vi "Execute Error Handling.vi"(8 "error in (no error)":errorcluster, 9 "Error":errorcluster, 10 "Error Level":T1, 11 "Interface Elevator in":refnum<class "Interface Elevator.lvclass">) -> (0 "error out":errorcluster, 3 "Interface Elevator out":refnum<class "Interface Elevator.lvclass">)   [LabVIEW 2022 SP3, in "Interface Elevator.lvclass"]
uses:
  Interface Elevator.lvclass
  Elevator Controller Actor/Elevator Controller Actor/Error Level.ctl
  Elevator Controller Actor/Elevator Controller Actor/Elevator Controller Actor.lvclass
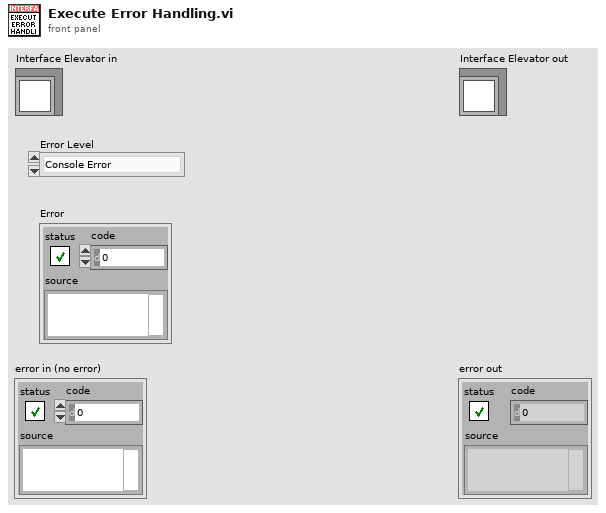
[diagram p1: front panel]
types:
  T1 = typedef "Elevator Controller Actor.lvlib/Elevator Controller Actor.lvclass/Error Level.ctl" = enum16{"Console Error", "Sensor Interface IO Error", "Process Step Error"}
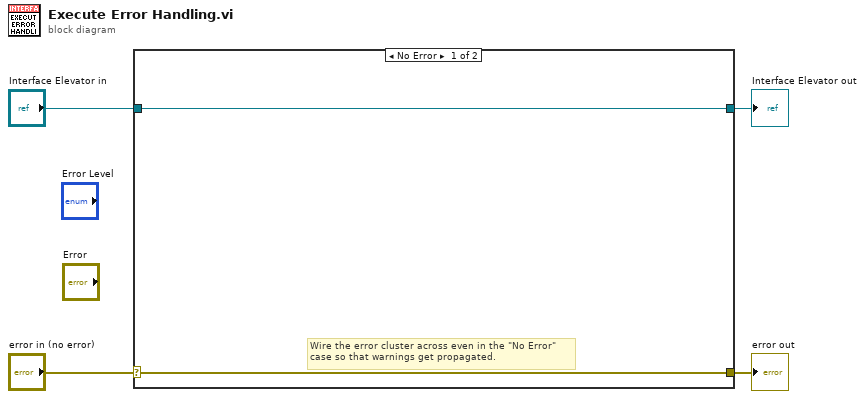
[diagram p0: block diagram]
diagram:
  n1 = case shown="No Error" "error in (no error)" {
    selector: "error in (no error)" -> [w5 w8]
    tunnel: [w5 w8] -> w3
    tunnel: [w6 w7] -> w1
    tunnel: "Interface Elevator in" -> [w6 w7]
    frame No Error {
      # "Wire the error cluster across even in the \"No Error\"\ncase so that warnings get propagated."
    }
    frame Error {
    }
  }
  "error out" <- w3
  "Interface Elevator out" <- w1
